vi "Create CellFormat.vi"(8 "error in":errorcluster, 11 "Formats":T1={"NumberFormatId"=164, "FontId"=0, "FillId"=0, "BorderId"=0, "FormatId"=0, "ApplyNumberFormat"=TRUE}) -> (0 "error out":errorcluster, 3 "CellFormat":refnum<k24>)   [LabVIEW 2019, in "Open Xml.lvlib"]
uses:
  Open Xml.lvlib
  D:/git/Open-Xml-LabVIEW/Source/DocumentFormat.OpenXml.dll
  DocumentFormat.OpenXml.dll
  D:/git/Open-Xml-LabVIEW/Source/DocumentFormat.OpenXml.Framework.dll
  DocumentFormat.OpenXml.Framework.dll
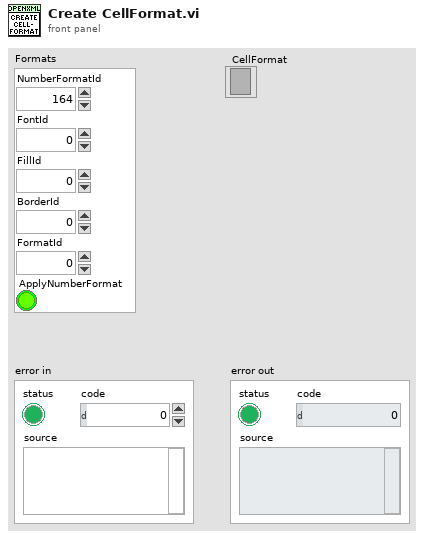
[diagram p1: front panel]
types:
  T1 = cluster{"NumberFormatId":u32, "FontId":u32, "FillId":u32, "BorderId":u32, "FormatId":u32, "ApplyNumberFormat":bool}
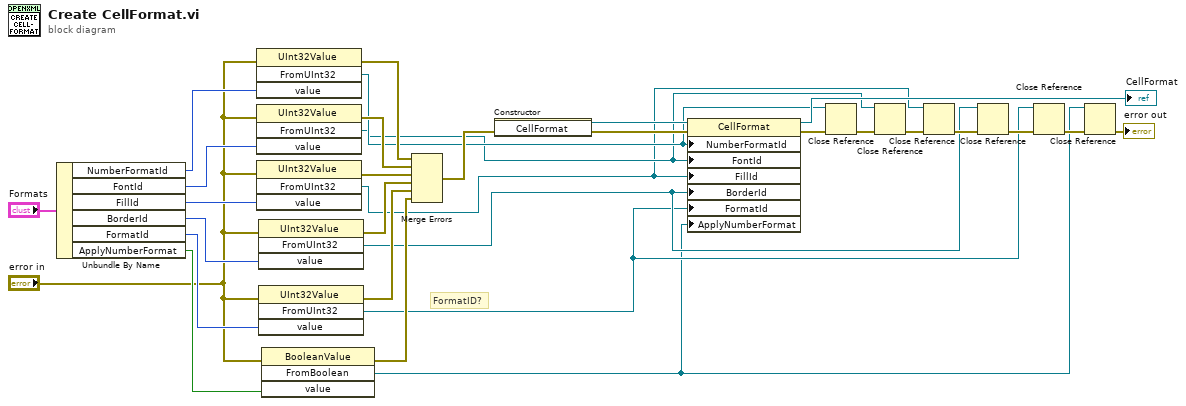
[diagram p0: block diagram]
diagram:
  # "FormatID?"
  n1 = Unbundle By Name("Formats") -> ("NumberFormatId"=w26:u32, "FontId"=w25:u32, "FillId"=w24:u32, "BorderId"=w23:u32, "FormatId"=w22:u32, "ApplyNumberFormat"=w21:bool)
  n2 = invoke class="UInt32Value" method="FromUInt32"(error in="error in", "value"=w26) -> (error out=w20:errorcluster, "FromUInt32"=w10:refnum<k24>)  [unwired: 2 in, 2 out]
  n3 = invoke class="UInt32Value" method="FromUInt32"(error in="error in", "value"=w25) -> (error out=w19:errorcluster, "FromUInt32"=w9:refnum<k24>)  [unwired: 2 in, 2 out]
  n4 = invoke class="UInt32Value" method="FromUInt32"(error in="error in", "value"=w24) -> (error out=w18:errorcluster, "FromUInt32"=w7:refnum<k24>)  [unwired: 2 in, 2 out]
  n5 = invoke class="UInt32Value" method="FromUInt32"(error in="error in", "value"=w23) -> (error out=w17:errorcluster, "FromUInt32"=w5:refnum<k24>)  [unwired: 2 in, 2 out]
  n6 = invoke class="UInt32Value" method="FromUInt32"(error in="error in", "value"=w22) -> (error out=w16:errorcluster, "FromUInt32"=w2:refnum<k24>)  [unwired: 2 in, 2 out]
  n7 = invoke class="BooleanValue" method="FromBoolean"(error in="error in", "value"=w21) -> (error out=w15:errorcluster, "FromBoolean"=w1:refnum<k24>)  [unwired: 2 in, 2 out]
  n8 = Merge Errors(w20, w19, w18, w17, w16, w15) -> (w14:errorcluster)
  n9 = constructor class="CellFormat"(error in=w14) -> (reference out=w29:refnum<k24>, error out=w30:errorcluster)  [unwired: 2 in, 1 out]
  n10 = property class="CellFormat"(reference=w29, error in=w30, "NumberFormatId"=w10, "FontId"=w9, "FillId"=w7, "BorderId"=w5, "FormatId"=w2, "ApplyNumberFormat"=w1) -> (reference out=→"CellFormat":refnum<k24>, error out=w27:errorcluster)
  n11 = Close Reference(reference=w10, error in (no error)=w27) -> (error out=w12:errorcluster)
  n12 = Close Reference(reference=w9, error in (no error)=w12) -> (error out=w11:errorcluster)
  n13 = Close Reference(reference=w7, error in (no error)=w11) -> (error out=w8:errorcluster)
  n14 = Close Reference(reference=w5, error in (no error)=w8) -> (error out=w6:errorcluster)
  n15 = Close Reference(reference=w2, error in (no error)=w6) -> (error out=w4:errorcluster)
  n16 = Close Reference(reference=w1, error in (no error)=w4) -> (error out=→"error out":errorcluster)
